vi "GenerateCode.vi"(1 "Terms":T1[](array[typedef]), 3 "Diagram":refnum<vi>, 5 "XRef":refnum<vi>, 6 "State In":T4={"Input Type"=variant(dbl 0.0), "Selection"=0, "Element Names"=[], "Type Strings"=[], "Element Types"=[]}) -> (0 "Generated Code?":bool, 2 "State Out":T4={"Input Type"=variant(dbl 0.0), "Selection"=0, "Element Names"=[], "Type Strings"=[], "Element Types"=[]}, 4 "Reply":string[](array[string]))   [LabVIEW 2015, in "Case-Tagged-Union.xnode"]
doc: "This ability VI is called when it is time to define the execution behavior of your XNode via LabVIEW's scripting API. This VI is only called when you have previously informed LabVIEW that you need to script through a GenerateCode reply. Diagram is a reference to a diagram of a temporary VI. This diagram contains exactly one front panel terminal for each terminal of your XNode. Terms is an array of pairs of Term IDs and terminal references. LabVIEW will copy code scripted into this diagram into your XNode and connect everything to the correct terminals. The front panel terminals that are on this diagram are special in that they can only be on the top level diagram.\n \n Generate Code? is used to tell LabVIEW whether or not you want to copy the scripted diagram over. If there is an error and you wish not to commit the changes, then the old XNode behavior will be left unchanged. If you set Generate Code? to false, then this VI will be called again next time type propagation is run. Otherwise, it will not be called until you indicate that it should be through the reply on another ability VI.\n \n Because the diagram you are scripting into is separate from the VI containing the XNode instance, type propagation and the data manager will run on the temporary VI after each scripting call.\n \n You should not use the Copy scripting method to move code into the temporary VI. This will adversely affect the user's clipboard. You should use the Move scripting method instead.\n\nDefault behavior: None.\n\nThis ability does not provide UI and OS messages are not handled.\n\nSee also: ModifyCode"
uses:
  Case-Tagged-Union.xnode
  State.ctl
  <vilib>/XNodeSupport/XNodeTermIDPair.ctl
  <vilib>/XNodeSupport/XNodeTermRef.ctl
  <vilib>/XNodeSupport/XNodeString.ctl
  <vilib>/Erdos Miller/LV-Scripting/LV-Scripting.lvlib
  <vilib>/XNodeSupport/NI_XNodeSupport.lvlib
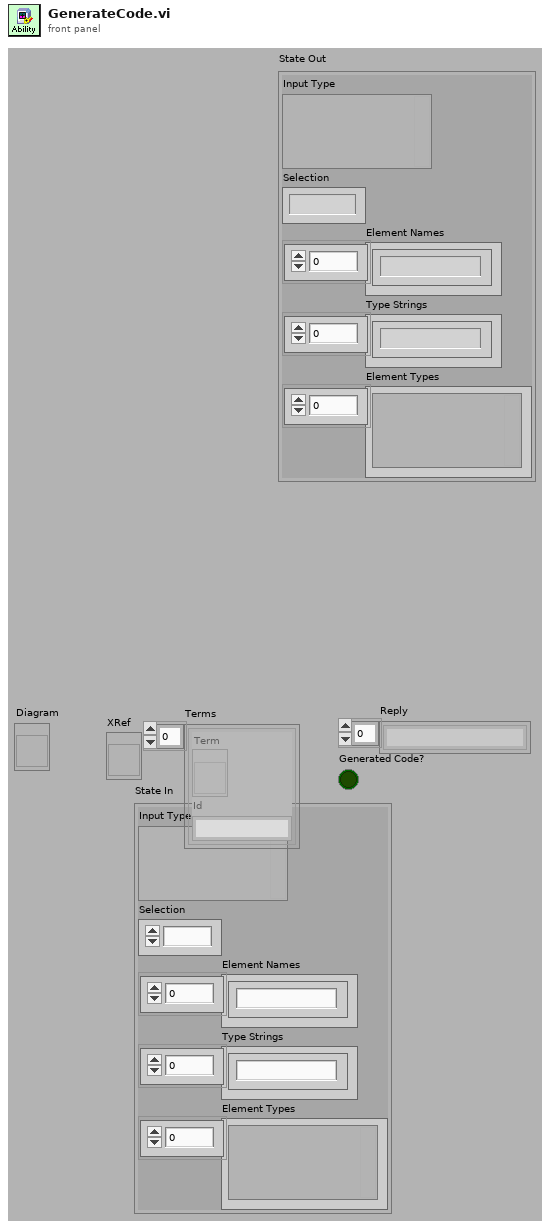
[diagram p1: front panel]
types:
  T1 = typedef "NI_XNodeSupport.lvlib/XNodeTermIDPair.ctl" = cluster{"Term":T2, "Id":T3}
  T2 = typedef "NI_XNodeSupport.lvlib/XNodeTermRef.ctl" = refnum<vi>
  T3 = typedef "NI_XNodeSupport.lvlib/XNodeString.ctl" = string
  T4 = typedef "Case-Tagged-Union.xnode/State.ctl" = cluster{"Input Type":variant, "Selection":i32, "Element Names":string[], "Type Strings":string[], "Element Types":variant[]}
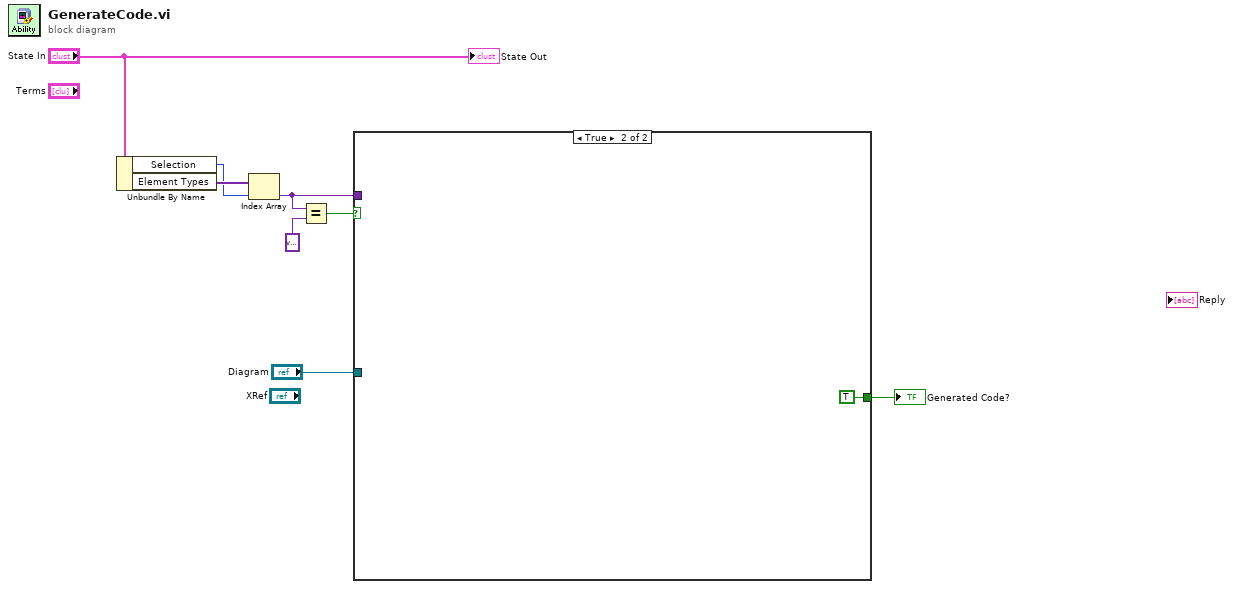
[diagram p0: block diagram]
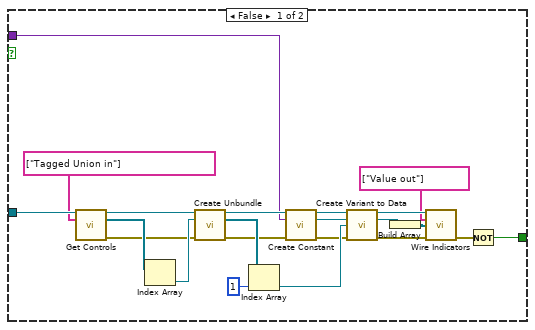
[diagram p2: hidden frame]
diagram:
  n1 = Unbundle By Name("State In") -> ("Selection"=w6:i32, "Element Types"=w7:variant[])
  n2 = Index Array(array=w7, index=w6) -> (element=w2:variant)
  n3 = Equal?(x=w2, y=variant) -> (x = y?=w4:bool)
  n4 = case shown="True" w4 {
    tunnel: "Diagram" -> [w30 _]
    tunnel: w2 -> [w21 _]
    tunnel: [w11 TRUE] -> w1
    frame False {
      n5 = call <vilib>:"Get Controls.vi"("Diagram in"=w30, "Control Names"=string[] ["Tagged Union in"]) -> ("Diagram out"=w27:refnum<vi>, "Control Terminals"=w28:refnum<vi>[], "error out"=w16:errorcluster)  [unwired: 11 in]
      n6 = Index Array(array=w28) -> (element=w26:refnum<vi>)  [unwired: 1 in]
      n7 = call <vilib>:"Create Unbundle.vi"("Diagram in"=w27, "input cluster"=w26, "error in (no error)"=w16) -> ("Diagram out"=w23:refnum<vi>, "Outputs"=w25:refnum<vi>[], "error out"=w17:errorcluster)  [unwired: 10 in]
      n8 = Index Array(array=w25, index=1) -> (element=w19:refnum<vi>)
      n9 = call <vilib>:"Create Constant.vi"("Diagram in"=w23, "Type"=w21, "error in (no error)"=w17) -> ("Diagram out"=w22:refnum<vi>, "Terminal"=w20:refnum<vi>, "error out"=w18:errorcluster)  [unwired: 10 in]
      n10 = call <vilib>:"Create Variant to Data.vi"("Diagram in"=w22, "type"=w20, "variant"=w19, "error in (no error)"=w18) -> ("Diagram out"=w15:refnum<vi>, "data"=w10:refnum<vi>, "error out"=w13:errorcluster)  [unwired: 8 in, 1 out]
      n11 = Build Array(w10) -> (w9:refnum<vi>[])
      n12 = call <vilib>:"Wire Indicators.vi"("Diagram in"=w15, "Indicator Names"=string[] ["Value out"], "Outputs"=w9, "error in (no error)"=w13) -> ("error out"=w12:errorcluster)  [unwired: 10 in, 1 out]
      n13 = Not(x=w12) -> (.not. x?=w11:bool)
    }
    frame True {
    }
  }
  "Generated Code?" <- w1
  "State Out" <- "State In"
